vi "RSZVB Load Calibration Kit.vi"(0 "VISA session":refnum<visa-resource-name>, 1 "File Name":string, 2 "Port Number 2 (1)":i32=1, 5 "Connector Name":string, 7 "Calibration Kit Name":string, 9 "Standard (0: Through (MM))":i32(ring) items=["Through (MM)"=0, "Through (FF)"=1, "Through (MF)"=2, "Line 1 (MM)"=3, "Line 1 (FF)"=4, "Line 1 (MF)"=5, "Offset short (M)"=7, "Offset short (F)"=8, "Attenuation (MM)"=9, "Attenuation (FF)"=10, "Attenuation (MF)"=11, "Symm Network (MM)"=12, "Symm Network (FF)"=13, "Symm Network (MF)"=14, "Open (M)"=15, "Open (F)"=16, "Short (M)"=17, "Short (F)"=18, "Reflect (M)"=19, "Reflect (F)"=20, "Match (M)"=21, "Match (F)"=22, "Sliding Match (M)"=23, "Sliding Match (F)"=24, "Line 2 (MM)"=25, "Line 2 (FF)"=26, "Line 2 (MF)"=27, "Line 3 (MM)"=28, "Line 3 (FF)"=29, "Line 3 (MF)"=30, "Offset short 2 (M)"=31, "Offset short 2 (F)"=32, "Offset short 3 (M)"=33, "Offset short 3 (F)"=34], 11 "error in (no error)":errorcluster {"code" format="%.0x"}, 12 "Port Number 1 (1)":i32=1, 13 "Calibration Kit Label":string) -> (4 "dup VISA session":refnum<visa-resource-name>, 15 "error out":errorcluster {"code" format="%.0x"})   [LabVIEW 2011]
doc: "This VI loads cal kit data for a specific connector type, cal kit, and calibration standard from a specified Touchstone file, assigning a label for the cal data. A restriction on the port assignment may be defined in addition.\n\nRemote-control command(s):\nMMEMory:LOAD:CKIT:SDATa '<conn_name>', '<ckit_name>', MMTHrough | MFTHrough | FFTHrough | MMLine | MMLINE1 | MMLINE2 | MMLINE3 | MFLine | MFLINE1 | MFLINE2 | MFLINE3 | FFLine | FFLINE1 | FFLINE2 | FFLINE3 | MMATten | MFATten | FFATten | MMSNetwork | MFSNetwork | FFSNetwork | MOPen | FOPen | MSHort | FSHort | MOSHort | MOSHORT1 | MOSHORT2 | MOSHORT3 | FOSHort | FOSHORT1 | FOSHORT2 | FOSHORT3 | MREFlect | FREFlect | MMTCh | FMTCh | MSMatch | FSMatch, '<stdlabel_name>', '<file_name>' [,<port1_no>][,<port2_no>]"
uses:
  _utility/RSZVB Global Data.vi
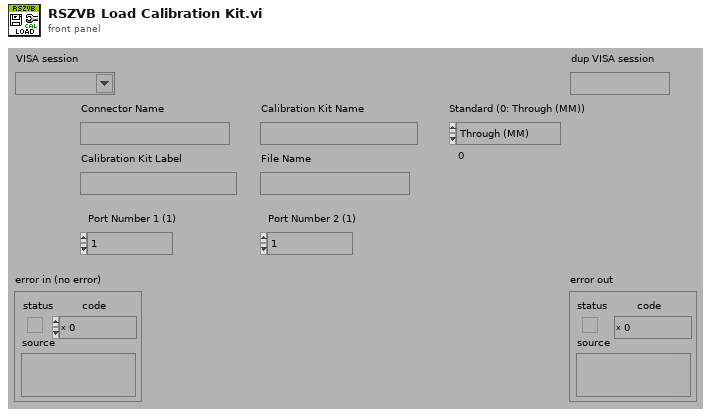
[diagram p1: front panel]
types:
  T1 = cluster{"Error Checking (T: On)":bool, "Installed Options":string[], "Data Valid?":bool, "Ports":i32, "Model":string[], "Option Checking (T: On)":bool}[]
  T2 = cluster{"Error Checking (T: On)":bool, "Installed Options":string[], "Data Valid?":bool, "Ports":i32, "Model":string[], "Option Checking (T: On)":bool}
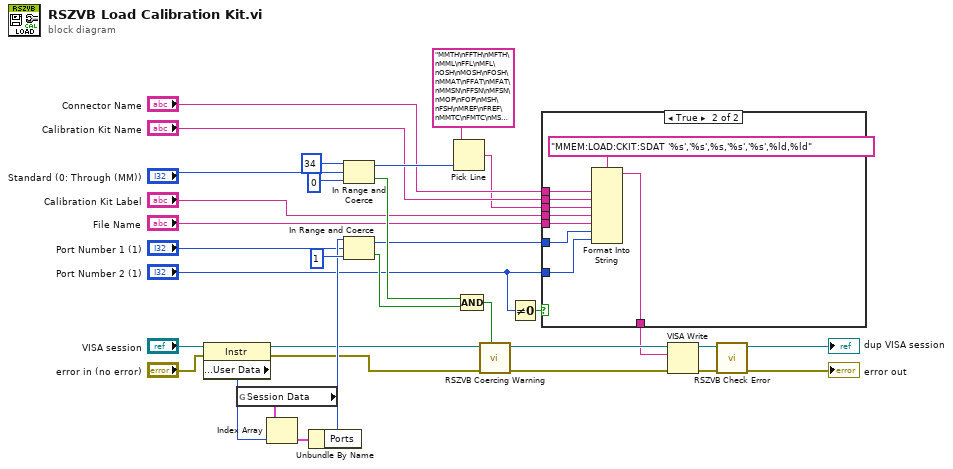
[diagram p0: block diagram]
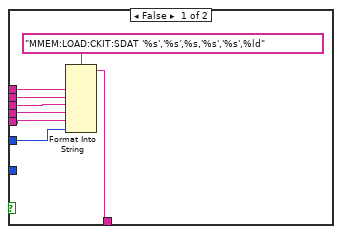
[diagram p2: hidden frame]
diagram:
  n1 = property class="Instr"(reference="VISA session", error in="error in (no error)") -> (reference out=w18:refnum<visa-resource-name>, error out=w19:errorcluster, "General Settings:User Data"=w24:u32)
  n2 = global read "RSZVB Global Data.vi" "Session Data"() -> (w25:T1)
  n3 = Index Array(array=w25, index=w24) -> (element=w26:T2)
  n4 = Unbundle By Name(w26) -> ("Ports"=w21:i32)
  n5 = In Range and Coerce(upper limit=34 ("lower limit"), x="Standard (0: Through (MM))", lower limit=0) -> (coerced(x)=w11:i32, In Range?=w13:bool)
  n6 = In Range and Coerce(upper limit=w21, x="Port Number 1 (1)", lower limit=1) -> (coerced(x)=w3:i32, In Range?=w12:bool)
  n7 = Pick Line(multi-line string="MMTH\nFFTH\nMFTH\nMML\nFFL\nMFL\nOSH\nMOSH\nFOSH\nMMAT\nFFAT\nMFAT\nMMSN\nFFSN\nMFSN\nMOP\nFOP\nMSH\nFSH\nMREF\nFREF\nMMTC\nFMTC\nMSM\nFSM\nMMLINE2\nFFLINE2\nMFLINE2\nMFLINE3\nFFLINE3\nMFLINE3\nMOSHORT2\nFOSHORT2\nMOSHORT3\nFOSHORT3", line index=w11) -> (output string=w6:string)  [unwired: 1 in]
  n8 = Compound Arithmetic op=AND(w13, w12) -> (w14:bool)
  n9 = call "RSZVB Coercing Warning.vi"("In Range?"=w14, "error in (no error)"=w19, "VISA session"=w18) -> ("error out"=w32:errorcluster, "dup VISA session"=w33:refnum<visa-resource-name>)  [unwired: 7 in]
  n10 = Not Equal To 0?(x="Port Number 2 (1)") -> (x != 0?=w1:bool)
  n11 = case shown="True" w1 {
    tunnel: [w41 w49] -> w28
    tunnel: "Connector Name" -> [w39 w48]
    tunnel: "Calibration Kit Name" -> [w38 w47]
    tunnel: w6 -> [w37 w46]
    tunnel: "Calibration Kit Label" -> [w36 w45]
    tunnel: "File Name" -> [w35 w44]
    tunnel: w3 -> [w34 w43]
    tunnel: "Port Number 2 (1)" -> [_ w42]
    frame False {
      n12 = Format Into String(format string="MMEM:LOAD:CKIT:SDAT '%s','%s',%s,'%s','%s',%ld", w39, w38, w37, w36, w35, w34) -> (resulting string=w41:string)  [unwired: 2 in, 1 out]
    }
    frame True {
      n13 = Format Into String(format string="MMEM:LOAD:CKIT:SDAT '%s','%s',%s,'%s','%s',%ld,%ld", w48, w47, w46, w45, w44, w43, w42) -> (resulting string=w49:string)  [unwired: 2 in, 1 out]
    }
  }
  n14 = VISA Write(VISA resource name=w33, write buffer=w28, error in (no error)=w32) -> (VISA resource name out=w30:refnum<visa-resource-name>, error out=w31:errorcluster)  [unwired: 1 out]
  n15 = call "RSZVB Check Error.vi"("error in (no error)"=w31, "VISA session"=w30) -> ("error out"=→"error out":errorcluster, "dup VISA session"=→"dup VISA session":refnum<visa-resource-name>)  [unwired: 8 in]
